vi "GetI_ITimerTimeout.vi"(0 "reference in":refnum<class "TimedDoor.lvclass">, 5 "error in (no error)":errorcluster) -> (14 "reference out":refnum<class "TimedDoor.lvclass">, 16 "InterfaceOut":refnum<class "ITimerTimeout.lvclass">, 19 "error out":errorcluster)   [LabVIEW 2020, in "TimedDoor.lvclass"]
doc: "Returns an Interaface that this class implements"
uses:
  TimedDoor.lvclass
  ITimerTimeout_Interface/ITimerTimeout.lvclass
  TimedDoor.lvclass/TimedDoor.ctl
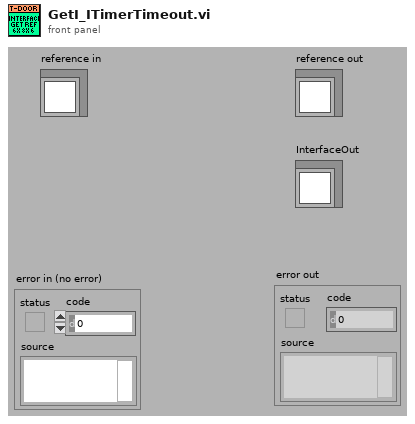
[diagram p1: front panel]
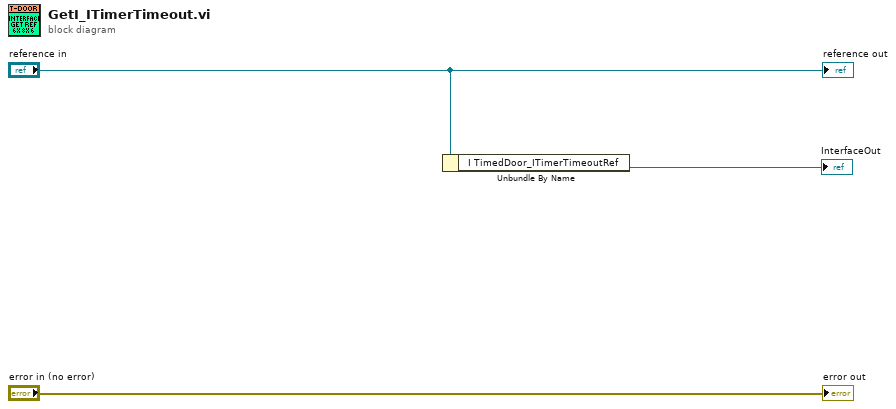
[diagram p0: block diagram]
diagram:
  n1 = Unbundle By Name("reference in") -> ("I TimedDoor_ITimerTimeoutRef"=→"InterfaceOut":refnum<class "ITimerTimeout.lvclass">)
  "error out" <- "error in (no error)"
  "reference out" <- "reference in"
